vi "GetBKValue.vi"(7 "Command":T1=enum."MaxVoltage", 8 "error in (no error)":errorcluster, 10 "Channel":string, 11 "Connection In":refnum<k5>) -> (0 "error out":errorcluster, 2 "Value":string, 3 "Connection Out":refnum<k5>)   [LabVIEW 2020]
uses:
  CommandTypeDef.ctl
panel:
  out "Sent Message":string
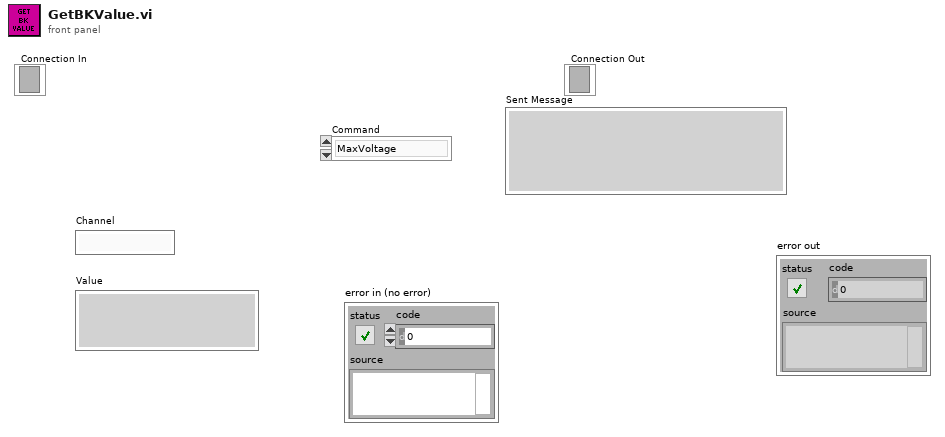
[diagram p1: front panel]
types:
  T1 = typedef "CommandTypeDef.ctl" = enum16{"Current", "MaxVoltage", "SlewRate", "EnableOutput", "Reset", "CurrentVoltage", "MaxCurrent"}
  T2 = enum16{"Standard", "Buffered", "CRLF", "Immediate"}
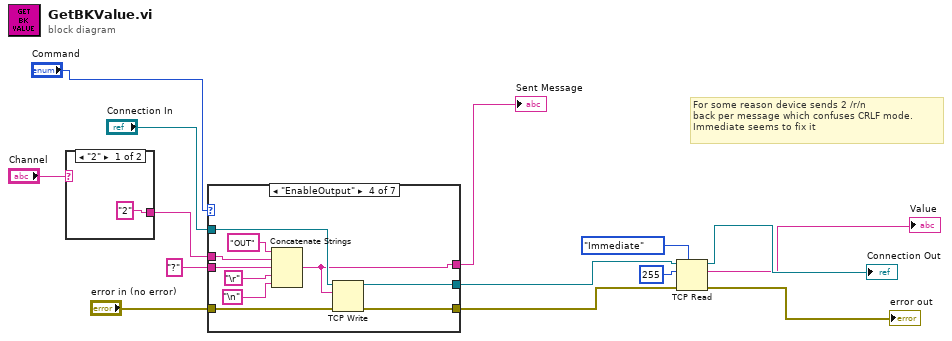
[diagram p0: block diagram]
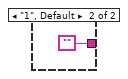
[diagram p2: hidden frame]
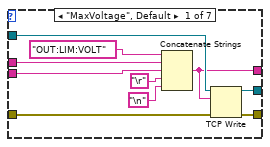
[diagram p3: hidden frame]
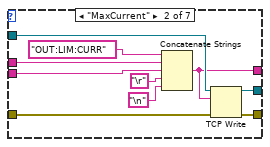
[diagram p4: hidden frame]
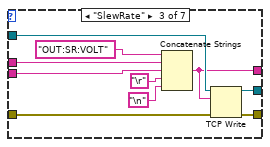
[diagram p5: hidden frame]
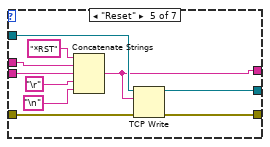
[diagram p6: hidden frame]
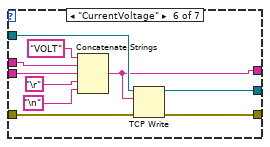
[diagram p7: hidden frame]
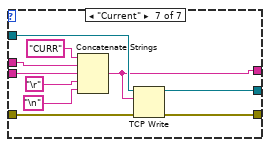
[diagram p8: hidden frame]
diagram:
  # "For some reason device sends 2 /r/n \nback per message which confuses CRLF mode. \nImmediate seems to fix it"
  n1 = case shown="\"2\"" "Channel" {
    tunnel: ["2" ""] -> w10
    frame "2" {
    }
    frame "1", Default {
    }
  }
  n2 = case shown="\"EnableOutput\"" "Command" {
    tunnel: "Connection In" -> [w23 w33 w43 w53 w63 w74 w84]
    tunnel: [w22 w32 w38 w48 w58 w73 w83] -> w3
    tunnel: [w21 w31 w39 w49 w59 w72 w82] -> w5
    tunnel: "error in (no error)" -> [w20 w30 w40 w50 w60 w71 w81]
    tunnel: w10 -> [w18 w28 w42 w52 w62 w69 w79]
    tunnel: "?" ("string") -> [w19 w29 w41 w51 w61 w67 w77]
    tunnel: [w17 w27 w37 w47 w57 w68 w78] -> w12
    frame "MaxVoltage", Default {
      n3 = Concatenate Strings("OUT:LIM:VOLT" ("data in"), w18, w19, "\r", "\n") -> (w17:string)
      n4 = TCP Write(connection ID=w23, data in=w17, error in (no error)=w20) -> (connection ID out=w22:refnum<k5>, error out=w21:errorcluster)  [unwired: 1 in, 1 out]
    }
    frame "MaxCurrent" {
      n5 = Concatenate Strings("OUT:LIM:CURR" ("data in"), w28, w29, "\r", "\n") -> (w27:string)
      n6 = TCP Write(connection ID=w33, data in=w27, error in (no error)=w30) -> (connection ID out=w32:refnum<k5>, error out=w31:errorcluster)  [unwired: 1 in, 1 out]
    }
    frame "SlewRate" {
      n7 = Concatenate Strings("OUT:SR:VOLT" ("data in"), w42, w41, "\r", "\n") -> (w37:string)
      n8 = TCP Write(connection ID=w43, data in=w37, error in (no error)=w40) -> (connection ID out=w38:refnum<k5>, error out=w39:errorcluster)  [unwired: 1 in, 1 out]
    }
    frame "EnableOutput" {
      n9 = Concatenate Strings("OUT" ("data in"), w52, w51, "\r", "\n") -> (w47:string)
      n10 = TCP Write(connection ID=w53, data in=w47, error in (no error)=w50) -> (connection ID out=w48:refnum<k5>, error out=w49:errorcluster)  [unwired: 1 in, 1 out]
    }
    frame "Reset" {
      n11 = Concatenate Strings("*RST" ("data in"), w62, w61, "\r", "\n") -> (w57:string)
      n12 = TCP Write(connection ID=w63, data in=w57, error in (no error)=w60) -> (connection ID out=w58:refnum<k5>, error out=w59:errorcluster)  [unwired: 1 in, 1 out]
    }
    frame "CurrentVoltage" {
      n13 = Concatenate Strings("VOLT" ("data in"), w69, w67, "\r", "\n") -> (w68:string)
      n14 = TCP Write(connection ID=w74, data in=w68, error in (no error)=w71) -> (connection ID out=w73:refnum<k5>, error out=w72:errorcluster)  [unwired: 1 in, 1 out]
    }
    frame "Current" {
      n15 = Concatenate Strings("CURR" ("data in"), w79, w77, "\r", "\n") -> (w78:string)
      n16 = TCP Write(connection ID=w84, data in=w78, error in (no error)=w81) -> (connection ID out=w83:refnum<k5>, error out=w82:errorcluster)  [unwired: 1 in, 1 out]
    }
  }
  "Sent Message" <- w12
  n17 = TCP Read(connection ID=w3, bytes to read=255, error in (no error)=w5, 7:T2."Immediate" ("mode (standard)")) -> (connection ID out=→"Connection Out":refnum<k5>, data out=→"Value":string, error out=→"error out":errorcluster)  [unwired: 1 in]
